vi "New Raw Message.vi"(8 "error in (no error)":errorcluster, 10 "Tags":T1(array[cluster]), 11 "Raw Message in":refnum<class "Raw Message.lvclass">) -> (0 "error out":errorcluster, 3 "Raw Message out":refnum<class "Raw Message.lvclass">)   [LabVIEW 2020, in "Protobuf RAW.lvlib" / "Raw Message.lvclass"]
uses:
  Raw Message.lvclass
  Tag/Basic Type.lvclass
  Raw Message.lvclass/Raw Message.ctl
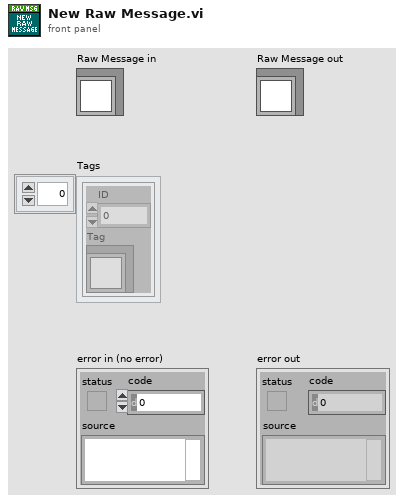
[diagram p1: front panel]
types:
  T1 = cluster{"ID":u32, "Tag":refnum<class "Basic Type.lvclass">}[]
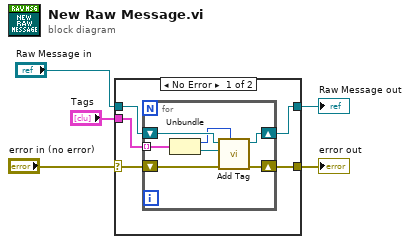
[diagram p0: block diagram]
diagram:
  n1 = case shown="No Error" "error in (no error)" {
    selector: "error in (no error)" -> [w10 w19]
    tunnel: [w9 w19] -> w4
    tunnel: [w7 w18] -> w2
    tunnel: "Raw Message in" -> [w8 w18]
    tunnel: "Tags" -> [w6 _]
    frame No Error {
      n2 = for {
        tunnel: w6 -> [w13] mode=indexing
        shift-right: [w16] -> w9
        shift-left: w10 -> [w17]
        shift-right: [w14] -> w7
        shift-left: w8 -> [w15]
        n3 = Unbundle(w13) -> ("ID"=w12:u32, "Tag"=w11:refnum<class "Basic Type.lvclass">)
        n4 = call-dynamic "Add Tag.vi"("ID"=w12, "error in (no error)"=w17, "Tag Value"=w11, "Message in"=w15) -> ("error out"=w16:errorcluster, "Message out"=w14:refnum<class "Raw Message.lvclass">)  [unwired: 6 in]
      }
    }
    frame Error {
    }
  }
  "error out" <- w4
  "Raw Message out" <- w2
